vi "HapticSTM_FBL.vi"() -> ()   [LabVIEW 2019]
uses:
  <userlib>/HapticSTM/HapticSTM.lvlib
  SubVIs/GlobalClicksHeight_FBL.vi
  <vilib>/sound2/lvsound2.llb/Sampling Mode.ctl
  <vilib>/sound2/lvsound2.llb/Sound Data Format.ctl
  <userlib>/Nanonis Prog Interface V5/Nanonis Prog Interface.lvlib
  <vilib>/sound2/lvsound2.llb/Sound Output Set Volume (Single).vi
  <vilib>/sound2/lvsound2.llb/Sound Output Write (DBL Single).vi
panel:
  in  "Scaling?":bool
  in  "Surface Location (nm)":dbl
  in  "Z Write?":bool
  in  "Planing?":bool
  in  "Plunge Depth (pm)":dbl=280.0 format="%.1f"
  out "Button":bool
  out "Setpoint (pA)":dbl
  in  "Maximum (pA)":dbl=9000.0
  out "Filtered Current (pA)":dbl format="%.1f"
  out "Current (pA)":dbl format="%.1f"
  out "Oy":dbl
  out "Ox":dbl
  out "W":dbl
  out "H":dbl
  out "Z Write (m)":dbl format="%^.1e"
  out "Z Read (m)":dbl format="%^#.1e"
  out "Vy":dbl format="%.1f"
  out "Vz":dbl format="%.1f"
  out "Vx":dbl format="%.1f"
  out "Fy":dbl format="%.1f"
  out "Fz":dbl format="%.1f"
  out "Fx":dbl format="%.1f"
  out "phi":dbl format="%.1f"
  out "psi":dbl format="%.1f"
  out "theta":dbl format="%.1f"
  out "x":dbl format="%.1f"
  out "y":dbl format="%.1f"
  out "z":dbl format="%0.1f"
  out "Height":dbl format="%^.1e"
  in  "Hardness":dbl=1.0 format="%.1f"
  in  "Mode":u16(ring) items=["Log w/ Exp Z", "Log w/ Lin Z"]
  in  "Reset Clicks":bool
  out "Clicks":i32
  in  "STOP":bool
  in  "START":bool
  out "Seq":i32
  out "SeqString":string
  out "Raw and Scaled Z Positions":cluster{dbl, "Y":dbl}(graph)
  out "Scaled Force and Current":T1(graph)
  in  "Sensitivity":dbl=1.0 format="%.1f"
  in  "Volume":dbl(slide)=50.0 scale=0.0..100.0
  in  "Device ID":u32
  # "Nanonis"
  # "Small"
  # "Large"
  # "No"
  # "Yes"
  # "Current"
  # "Frame"
  # "Z Controller"
  # "Haptic Pen"
  # "Position"
  # "Force"
  # "Angles"
  # "Velocity"
  # "Surface"
  # "Clicks"
  # "Haptic STM Controller 3000"
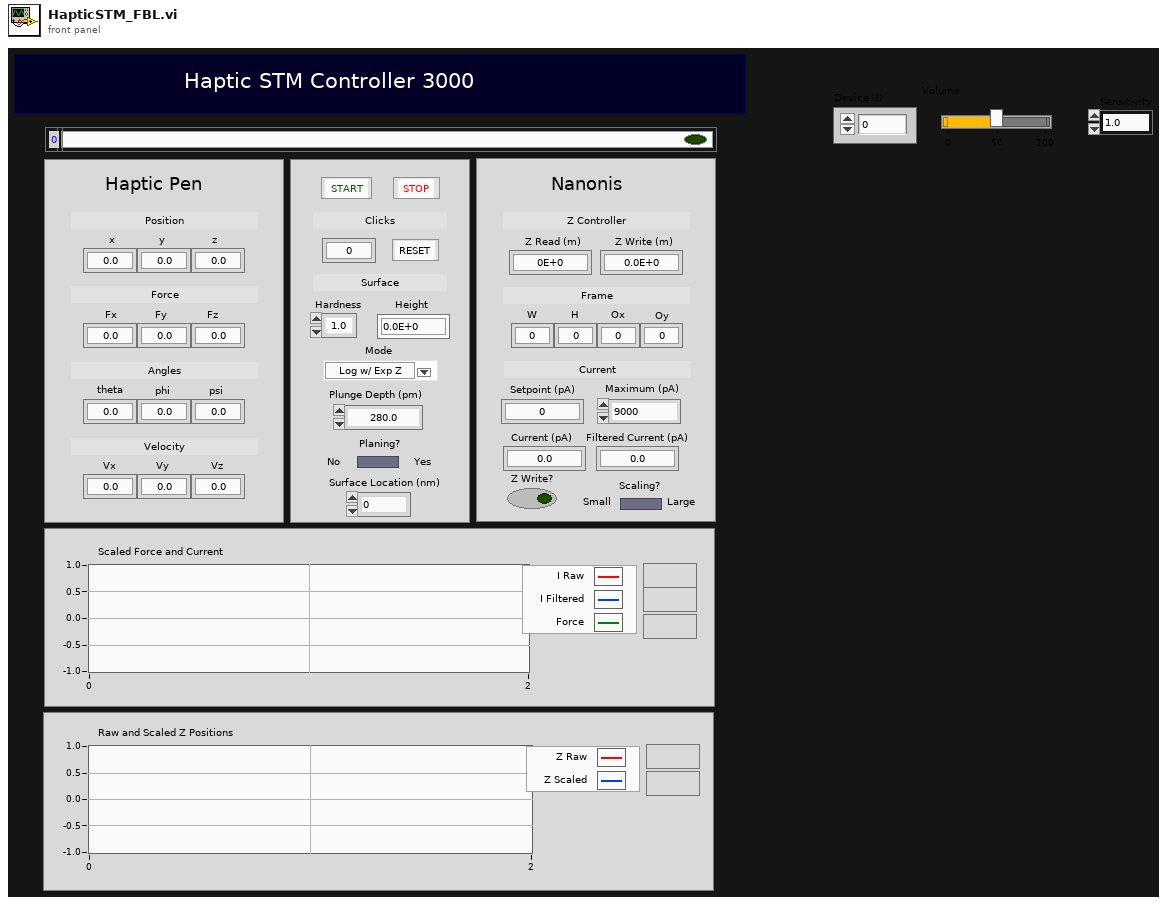
[diagram p1: front panel]
types:
  T1 = cluster{"Current (pA)":sgl, "Filtered Current (pA)":dbl, dbl}
  T2 = typedef "Sound Data Format.ctl" = cluster{"sample rate (S/s)":dbl, "number of channels":i32, "bits per sample":i32}
  T3 = typedef "Sampling Mode.ctl" = i32
  T4 = typedef "Sound Output Task ID.ctl" = u32
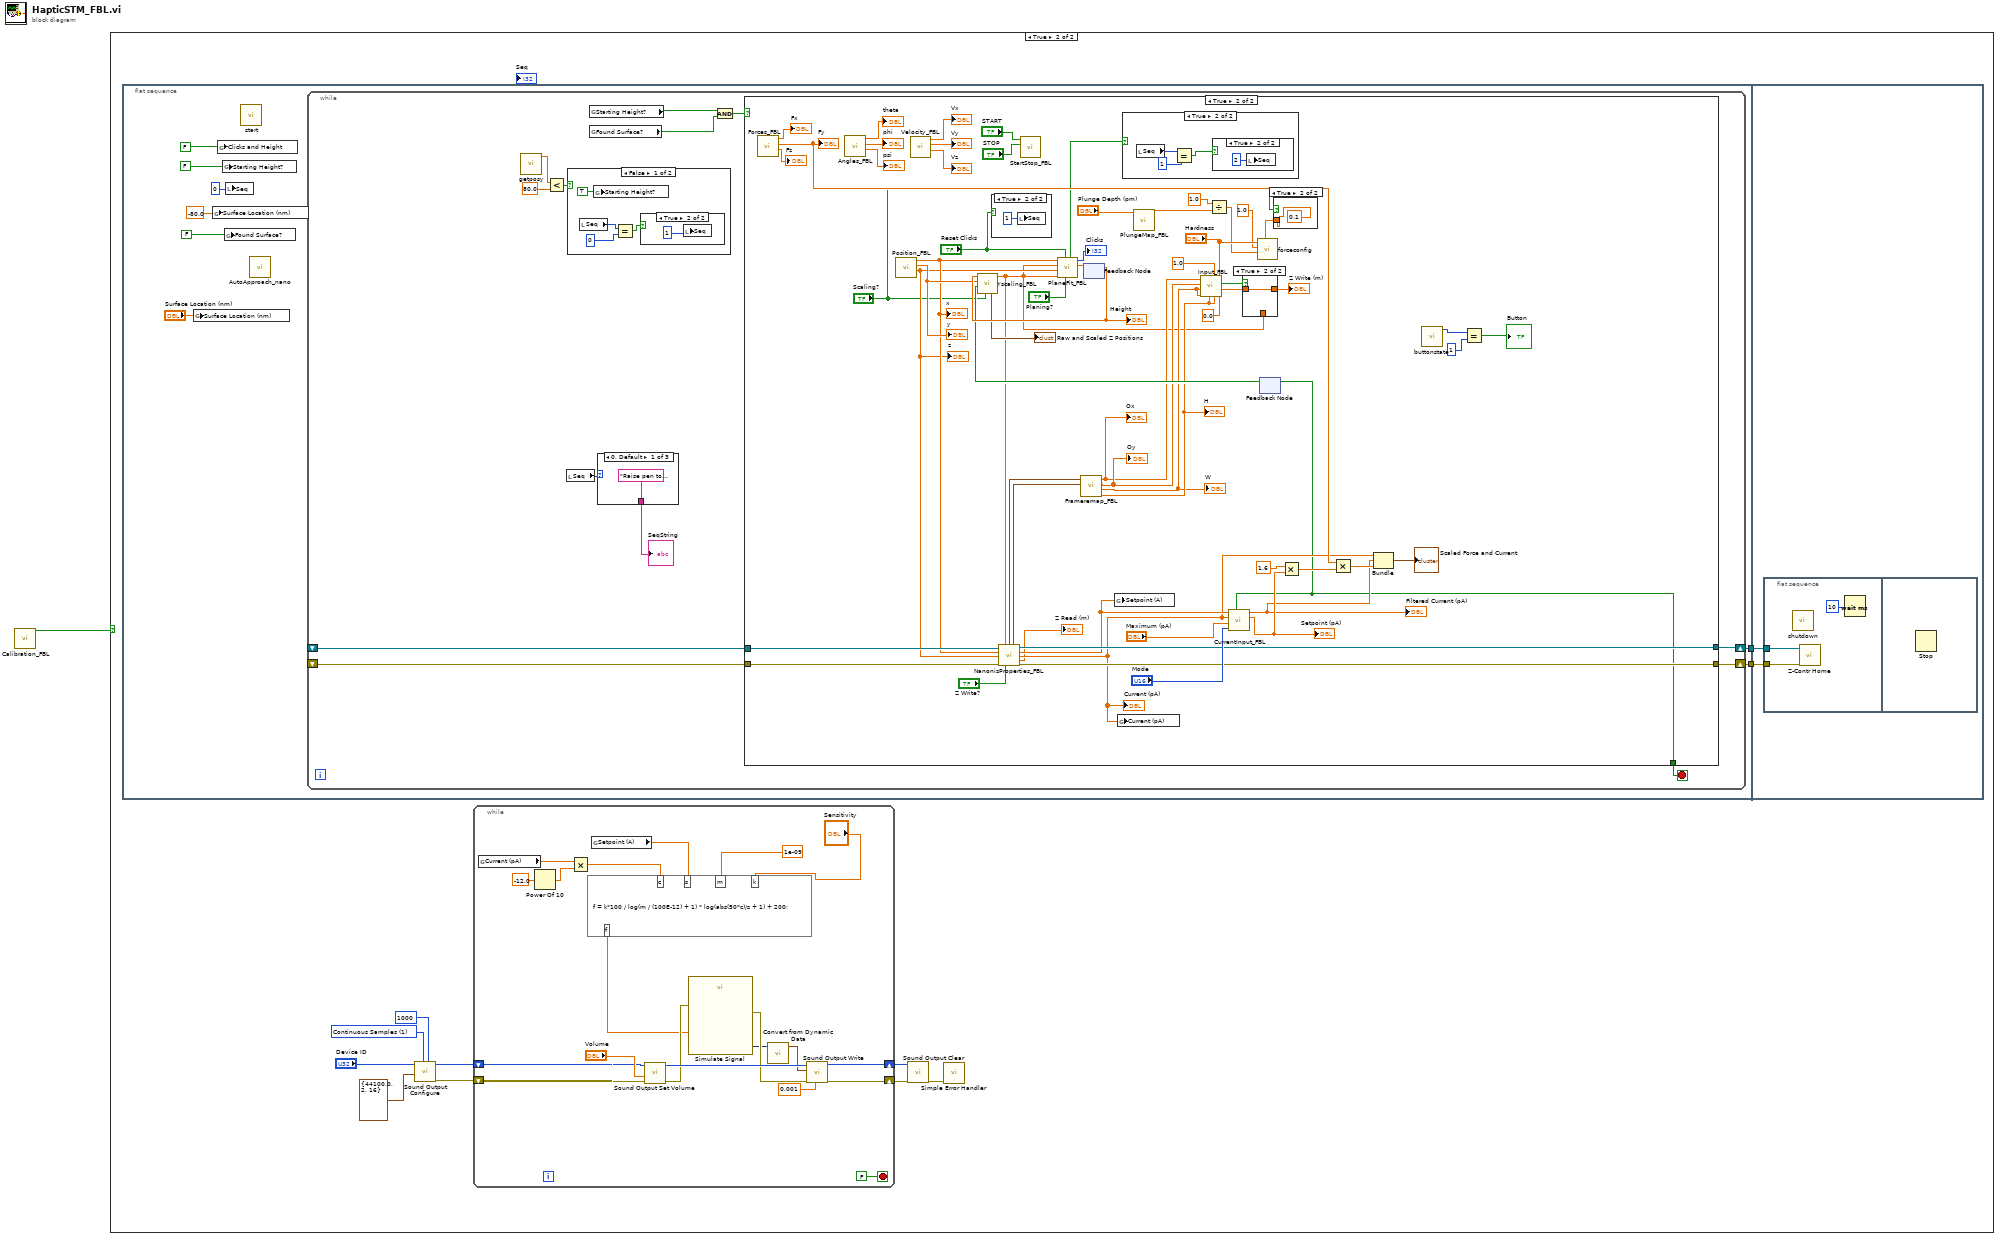
[diagram p0: block diagram]
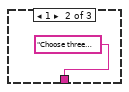
[diagram p3: hidden frame]
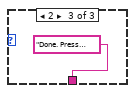
[diagram p4: hidden frame]
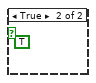
[diagram p6: hidden frame]
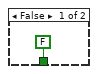
[diagram p7: hidden frame]
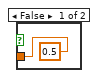
[diagram p8: hidden frame]
diagram:
  n1 = call "Calibration_FBL.vi"() -> ("Calibration Complete?"=w1:bool)  [unwired: 11 in]
  n2 = case shown="True" w1 {
    frame False {
    }
    frame True {
      w11 = T3 1 items=["Finite Samples", "Continuous Samples"] ("sample mode")
      n3 = flat-sequence {
        tunnel: [w14] -> w3
        tunnel: [w13] -> w2
        tunnel: w3 -> [w115]
        tunnel: w2 -> [w114]
        frame #0 {
          n4 = global write "GlobalClicksHeight_FBL.vi" "Surface Location (nm)"("Surface Location (nm)") -> ()
          n5 = global write "GlobalClicksHeight_FBL.vi" "Surface Location (nm)"(-80.0 ("Surface Location")) -> ()
          n6 = global write "GlobalClicksHeight_FBL.vi" "Clicks and Height"(FALSE ("Clicks and Height")) -> ()
          n7 = global write "GlobalClicksHeight_FBL.vi" "Starting Height?"(FALSE ("Clicks and Height")) -> ()
          n8 = global write "GlobalClicksHeight_FBL.vi" "Found Surface?"(FALSE ("Clicks and Height")) -> ()
          n9 = local write "Seq"(0 ("Seq")) -> ()
          n10 = call <userlib>:"start.vi"() -> ()  [unwired: 11 in, 1 out]
          n11 = call "AutoApproach_nano.vi"() -> ()  [unwired: 12 in]
          n12 = while {
            shift-right: [w24] -> w13
            shift-left: _ -> [w25]
            shift-right: [w23] -> w14
            shift-left: _ -> [w22]
            stop <- w21 stop-if-true
            n13 = call <userlib>:"getposy.vi"() -> ("function return"=w33:dbl)  [unwired: 11 in]
            n14 = Less?(x=w33, y=80.0) -> (x < y?=w31:bool)
            n15 = local read "Seq"() -> (w30:i32)
            n16 = case shown="False" w31 {
              frame False {
                n17 = local read "Seq"() -> (w39:i32)
                n18 = global write "GlobalClicksHeight_FBL.vi" "Starting Height?"(TRUE ("Starting Height?")) -> ()
                n19 = Equal?(x=w39, y=0) -> (x = y?=w37:bool)
                n20 = case shown="True" w37 {
                  frame False {
                  }
                  frame True {
                    n21 = local write "Seq"(1 ("Seq")) -> ()
                  }
                }
              }
              frame True {
                (unwired) TRUE ("Clicks and Height")
              }
            }
            n22 = global read "GlobalClicksHeight_FBL.vi" "Starting Height?"() -> (w27:bool)
            n23 = global read "GlobalClicksHeight_FBL.vi" "Found Surface?"() -> (w26:bool)
            n24 = case shown="0, Default" w30 {
              tunnel: ["Raise pen to begin." "Choose three points, then raise the arm to plane." "Done. Press 'STOP' to stop at anytime."] -> w29
              frame 0, Default {
              }
              frame 1 {
              }
              frame 2 {
              }
            }
            "SeqString" <- w29
            n25 = And(x=w27, y=w26) -> (x .and. y?=w28:bool)
            n26 = case shown="True" w28 {
              tunnel: w25 -> [_ w60]
              tunnel: [_ w59] -> w24
              tunnel: [_ w58] -> w23
              tunnel: w22 -> [_ w57]
              tunnel: [FALSE ("Current Maxed?") w45] -> w21
              frame False {
              }
              frame True {
                n27 = call "Forces_FBL.vi"() -> ("Fz"=→"Fz":dbl, "Fy"=w89:dbl, "Fx"=→"Fx":dbl)  [unwired: 9 in]
                "Fy" <- w89
                n28 = call "Angles_FBL.vi"() -> ("psi"=→"psi":dbl, "phi"=→"phi":dbl, "theta"=→"theta":dbl)  [unwired: 9 in]
                n29 = call "Position_FBL.vi"() -> ("Z"=w55:dbl, "Y"=w85:dbl, "X"=w56:dbl)  [unwired: 9 in]
                "x" <- w56
                "y" <- w85
                "z" <- w55
                n30 = call "Velocity_FBL.vi"() -> ("VZ"=→"Vz":dbl, "VY"=→"Vy":dbl, "VX"=→"Vx":dbl)  [unwired: 9 in]
                n31 = case shown="True" "Reset Clicks" {
                  frame False {
                  }
                  frame True {
                    n32 = local write "Seq"(1 ("Seq")) -> ()
                  }
                }
                n33 = call "StartStop_FBL.vi"("STOP"="STOP", "START"="START") -> ()  [unwired: 10 in]
                n34 = feedback #1() -> (w92:dbl)  [unwired: 1 in]
                "Height" <- w92
                n35 = call "PlungeMap_FBL.vi"("Input (pA)"="Plunge Depth (pm)") -> ("output"=w47:dbl)  [unwired: 10 in]
                n36 = Divide(x=1.0, y=w47) -> (x/y=w70:dbl)
                n37 = feedback #2() -> (w91:bool)  [unwired: 1 in]
                n38 = call "Yscaling_FBL.vi"("Scaling?"="Scaling?", "Current Maxed?"=w91, "Y"=w85, "Plane Height"=w92) -> ("y scaled (m)"=w51:dbl, "Zpos Graph (nm)"=→"Raw and Scaled Z Positions":cluster{dbl, "function return":dbl})  [unwired: 6 in]
                n39 = call "NanonisProperties_FBL.vi"("Application reference"=w57, "Z Write (m)"=w51, "X pen (nm)"=w56, "Z pen (nm)"=w55, "Error in"=w60, "Z Write?"="Z Write?") -> ("Frame Size (m)"=w49:cluster{"Width":sgl, "Height":sgl}, "Frame Origin (m)"=w50:cluster{"Xc":sgl, "Yc":sgl}, "Application ref out"=w58:refnum<vi>, "Setpoint (A)"=w54:sgl, "Current (pA)"=w53:sgl, "Z Read (m)"=→"Z Read (m)":sgl, "error out"=w59:errorcluster)  [unwired: 3 in]
                "Current (pA)" <- w53
                n40 = call "PlaneFit_FBL.vi"("Planing y/n?"="Planing?", "Reset Clicks"="Reset Clicks", "Y PEN"=w51, "Z"=w55, "Nano Z"=w51, "X"=w56) -> ("Plane Height (m)"=w93:dbl, "Clicks"=→"Clicks":i32, "Planing Done?"=w78:bool)  [unwired: 3 in]
                n41 = call "Frameremap_FBL.vi"("Frame Origin (m)"=w50, "Frame Size (m)"=w49) -> ("FH"=w69:dbl, "FW"=w68:dbl, "Z Origin"=w67:dbl, "X Origin"=w66:dbl)  [unwired: 6 in]
                "H" <- w69
                "W" <- w68
                "Ox" <- w66
                "Oy" <- w67
                n42 = feedback-in #1(w93) -> ()
                n43 = global write "GlobalClicksHeight_FBL.vi" "Setpoint (A)"(w54) -> ()
                n44 = global write "GlobalClicksHeight_FBL.vi" "Current (pA)"(w53) -> ()
                n45 = case shown="True" w78 {
                  frame False {
                  }
                  frame True {
                    n46 = local read "Seq"() -> (w112:i32)
                    n47 = Equal?(x=w112, y=1) -> (x = y?=w110:bool)
                    n48 = case shown="True" w110 {
                      frame False {
                      }
                      frame True {
                        n49 = local write "Seq"(2 ("Seq")) -> ()
                      }
                    }
                  }
                }
                n50 = call "Input_FBL.vi"("Current * 10^input"=0.0, "Sensitivity"="Hardness", "Scopez"=w69, "Drag"=1.0, "FH"=w69, "FW"=w68, "Scopex"=w68, "Z origin"=w67, "X origin"=w66) -> ("Scaled Current"=w72:dbl, "feedback"=w74:bool)  [unwired: 1 in]
                n51 = call "CurrentInput_FBL.vi"("Mode"="Mode", "Maximum (pA)"="Maximum (pA)", "Current (pA)"=w53, "Setpoint (A)"=w54) -> ("Setpoint (pA)"=w62:dbl, "Filtered Current (pA)"=w61:dbl, "Current Maxed?"=w45:bool)  [unwired: 5 in]
                "Filtered Current (pA)" <- w61
                "Setpoint (pA)" <- w62
                n52 = case shown="True" w74 {
                  tunnel: [w107 w108] -> w73
                  tunnel: w72 -> [_ w108]
                  tunnel: w51 -> [w107 _]
                  frame False {
                  }
                  frame True {
                  }
                }
                "Z Write (m)" <- w73
                n53 = feedback-in #2(w45) -> ()
                n54 = case shown="True" "Scaling?" {
                  tunnel: [0.5 0.1] -> w44
                  frame False {
                  }
                  frame True {
                  }
                }
                n55 = call <userlib>:"forceconfig.vi"("spc"=w44, "c"=w70, "b"=1.0, "a"="Hardness") -> ()  [unwired: 8 in]
                n56 = Multiply(x=1.6 ("y"), y=w62) -> (x*y=w86:dbl)
                n57 = Multiply(x=w89, y=w86) -> (x*y=w88:dbl)
                n58 = Bundle("Current (pA)"=w53, "Filtered Current (pA)"=w61, w88) -> (→"Scaled Force and Current":T1)  [unwired: 1 in]
                n59 = call <userlib>:"buttonstate.vi"() -> ("function return"=w84:i32)  [unwired: 11 in]
                n60 = Equal?(x=w84, y=1) -> (x = y?=→"Button":bool)
              }
            }
          }
        }
        frame #1 {
          n61 = flat-sequence {
            tunnel: w115 -> [w118]
            tunnel: w114 -> [w117]
            frame #0 {
              n62 = call <userlib>:"shutdown.vi"() -> ()  [unwired: 12 in]
              n63 = call <userlib>:"Z-Contr Home.vi"("Error in (no error)"=w117, "Application ref in"=w118) -> ()  [unwired: 8 in, 2 out]
              n64 = Wait (ms)(milliseconds to wait=u32 10) -> ()  [unwired: 1 out]
            }
            frame #1 {
              n65 = Stop() -> ()  [unwired: 1 in]
            }
          }
        }
      }
      n66 = call <vilib>:"Sound Output Configure.vi"("number of samples/ch"=1000 ("Number of Samples/ch"), "sample mode"=w11, "sound format"=T2 {"sample rate (S/s)"=44100.0, "number of channels"=2, "bits per sample"=16} ("Sound Format"), "device ID"="Device ID") -> ("error out"=w7:errorcluster, "task ID"=w8:T4)  [unwired: 6 in]
      n67 = while {
        shift-right: [w130] -> w6
        shift-left: w8 -> [w132]
        shift-right: [w129] -> w5
        shift-left: w7 -> [w131]
        stop <- FALSE stop-if-true
        n68 = global read "GlobalClicksHeight_FBL.vi" "Current (pA)"() -> (w121:dbl)
        n69 = Power Of 10(x=-12.0) -> (10^x=w123:dbl)
        n70 = Multiply(x=w121, y=w123) -> (x*y=w120:dbl)
        n71 = global read "GlobalClicksHeight_FBL.vi" "Setpoint (A)"() -> (w125:dbl)
        n72 = formula code="f = k*100 / log(m / (100E-12) + 1) * log(abs(50*c)/s + 1) + 200;"("c"=w120, "m"=1e-09 ("input variable"), "s"=w125, "k"="Sensitivity") -> ("f"=w124:dbl)
        n73 = call-poly <vilib>:"Sound Output Set Volume.vi"("error in (no error)"=w131, "volume"="Volume", "task ID"=w132) -> ("error out"=w135:errorcluster, "task ID out"=w138:T4)  [unwired: 7 in]
        n74 = call "Simulate Signal"("Frequency"=w124, "error in (no error)"=w135) -> ("Sine"=w133:dynamicdata, "error out"=w134:errorcluster)  [unwired: 12 in]
        n75 = call "Convert from Dynamic Data"("Dynamic Data Type"=w133) -> ("Waveform"=w136:waveform(dbl))  [unwired: 3 in]
        n76 = call-poly <vilib>:"Sound Output Write.vi"("timeout (sec)"=0.001, "error in (no error)"=w134, "data"=w136, "task ID"=w138) -> ("error out"=w129:errorcluster, "task ID out"=w130:T4)  [unwired: 6 in]
      }
      n77 = call <vilib>:"Sound Output Clear.vi"("error in (no error)"=w5, "task ID"=w6) -> ("error out"=w10:errorcluster)  [unwired: 9 in]
      n78 = call <vilib>:"Simple Error Handler.vi"("error in (no error)"=w10) -> ()  [unwired: 4 in, 5 out]
    }
  }
